vi "Obtain Sheet.vi"(6 "Create if non-existant? (T)":bool=TRUE, 8 "error in (no error)":errorcluster, 10 "Sheet Name":string, 11 "ooCalc in":refnum<class "ooCalc.lvclass">) -> (0 "error out":errorcluster, 2 "Sheet":refnum<k24>, 3 "ooCalc out":refnum<class "ooCalc.lvclass">)   [LabVIEW 2009, in "ooCalc.lvclass"]
uses:
  ooCalc.lvclass
  C:/Projets/LAVAG/OpenOfficeRGT/AODL/DLLs/AODL.dll
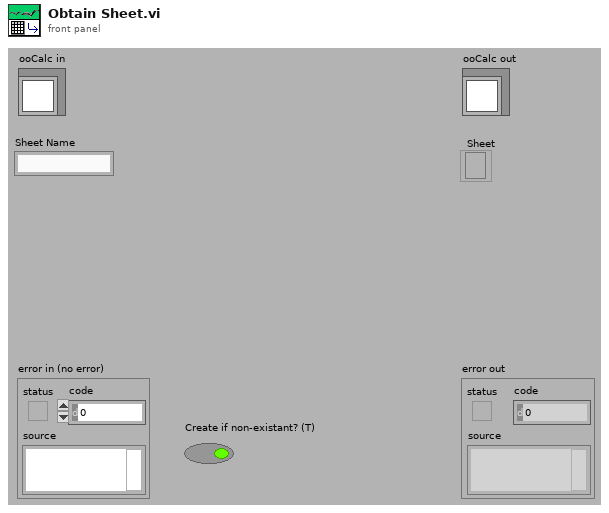
[diagram p1: front panel]
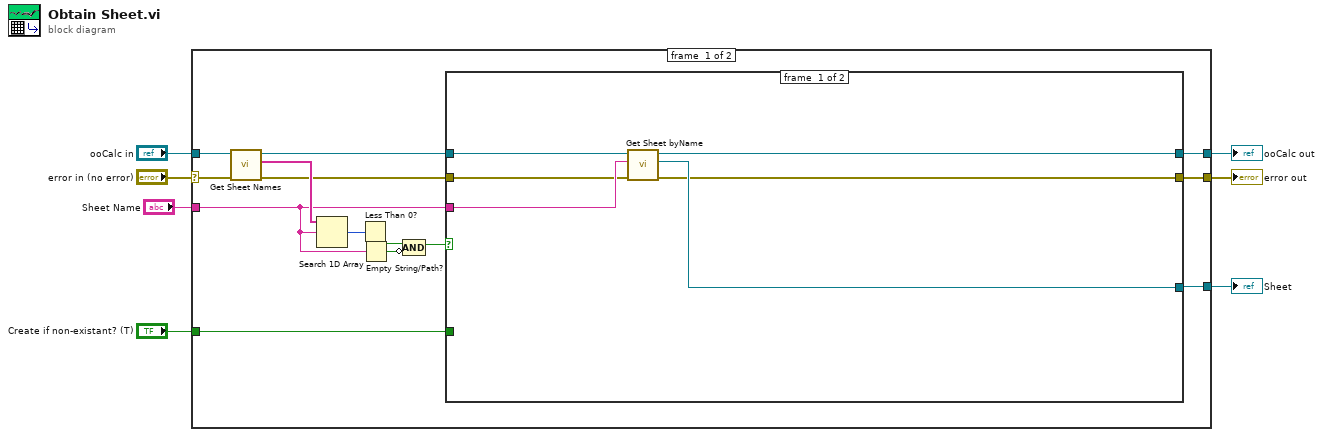
[diagram p0: block diagram]
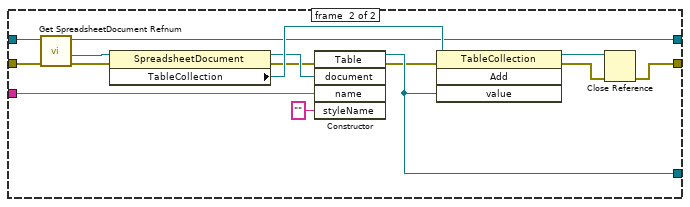
[diagram p3: hidden frame]
diagram:
  n1 = case shown="No Error" "error in (no error)" {
    selector: "error in (no error)" -> [w10 w53]
    tunnel: [w15 w53] -> w6
    tunnel: [w11 w52] -> w4
    tunnel: "ooCalc in" -> [w13 w52]
    tunnel: [w21 _] -> w3
    tunnel: "Sheet Name" -> [w19 _]
    tunnel: "Create if non-existant? (T)" -> [w8 _]
    frame #0 {
      n2 = call "Get Sheet Names.vi"("error IO"=w10, "ooCalc in"=w13) -> ("error out"=w9:errorcluster, "Sheets"=w20:string[], "ooCalc out"=w12:refnum<class "ooCalc.lvclass">)  [unwired: 7 in]
      n3 = Search 1D Array(1D array=w20, element=w19) -> (index of element=w14:i32)  [unwired: 1 in]
      n4 = Less Than 0?(x=w14) -> (x < 0?=w18:bool)
      n5 = Empty String/Path?(string/path=w19) -> (empty?=w17:bool)
      n6 = Compound Arithmetic op=AND(w18, invert w17) -> (w16:bool)
      n7 = case shown="True" w16 {
        tunnel: [w24 w32] -> w21
        tunnel: w19 -> [w26 w34]
        tunnel: w9 -> [w23 w31]
        tunnel: [w22 w30] -> w15
        tunnel: w12 -> [w27 w33]
        tunnel: [w25 w28] -> w11
        tunnel: w8 -> [_ w29]
        frame #0 {
          n8 = call "Get Sheet byName.vi"("error IO"=w23, "SheetName"=w26, "ooCalc in"=w27) -> ("error out"=w22:errorcluster, "Sheet"=w24:refnum<k24>, "ooCalc out"=w25:refnum<class "ooCalc.lvclass">)  [unwired: 6 in]
        }
        frame #1 {
          n9 = case shown="True" w29 {
            tunnel: w34 -> [_ w51]
            tunnel: w33 -> [w36 w40]
            tunnel: [_ w48] -> w32
            tunnel: w31 -> [w35 w38]
            tunnel: [w35 w44] -> w30
            tunnel: [w36 w39] -> w28
            frame #0 {
            }
            frame #1 {
              n10 = call-dynamic "Get SpreadsheetDocument Refnum.vi"("error in (no error)"=w38, "ooCalc in"=w40) -> ("error out"=w37:errorcluster, "SpreadsheetDocument"=w41:refnum<k24>, "ooCalc out"=w39:refnum<class "ooCalc.lvclass">)  [unwired: 7 in]
              n11 = property on="Property Node" class="SpreadsheetDocument"(reference=w41, error in=w37) -> (reference out=w47:refnum<k24>, error out=w46:errorcluster, "TableCollection"=w49:refnum<k24>)
              n12 = constructor class="Table"(error in=w46, "document"=w47, "name"=w51, "styleName"="") -> (reference out=w48:refnum<k24>, error out=w45:errorcluster)  [unwired: 2 in, 4 out]
              n13 = invoke class="TableCollection" method="Add"(reference=w49, error in=w45, "value"=w48) -> (reference out=w43:refnum<k24>, error out=w42:errorcluster)  [unwired: 1 in, 2 out]
              n14 = Close Reference(reference=w43, error in (no error)=w42) -> (error out=w44:errorcluster)
            }
          }
        }
      }
    }
    frame #1 {
    }
  }
  "error out" <- w6
  "ooCalc out" <- w4
  "Sheet" <- w3
